vi "mainActivity__viRemove.vi"(8 "error in":errorcluster, 11 "VI":path) -> (0 "error out":errorcluster)   [LabVIEW 2014]
uses:
  glb/glb_static.vi
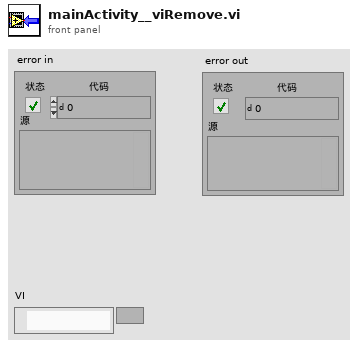
[diagram p1: front panel]
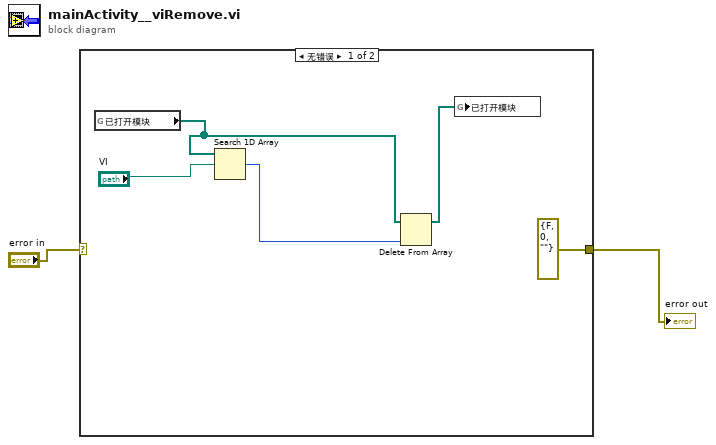
[diagram p0: block diagram]
diagram:
  n1 = case shown="无错误" "error in" {
    selector: "error in" -> [_ w8]
    tunnel: [errorcluster {"status"=FALSE, "code"=0, "source"=""} ("45002") w8] -> w1
    frame No Error {
      n2 = global read "glb_static.vi" "已打开模块"() -> (w4:path[])
      n3 = Search 1D Array(1D array=w4, element="VI") -> (index of element=w6:i32)  [unwired: 1 in]
      n4 = Delete From Array(array=w4, index=w6) -> (array with subset deleted=w3:path[])  [unwired: 1 in, 1 out]
      n5 = global write "glb_static.vi" "已打开模块"(w3) -> ()
    }
    frame Error {
    }
  }
  "error out" <- w1
